vi "PickOffensiveRobots_v2.vi"(0 "object in":refnum<class "Game.lvclass">, 2 "GameRef":refnum<data-value>, 5 "error in (no error)":errorcluster) -> (14 "object out":refnum<class "Game.lvclass">, 19 "error out":errorcluster)   [LabVIEW 2023, in "Game.lvclass"]
uses:
  Game.lvclass
  Game.lvclass/Game.ctl
  Team_class/Team.lvclass/Team.ctl
  Team_class/Write RobotRef.vi
  Ally_class/Ally.lvclass
  C:/Users/ebert/Documents/codes/SSL/repo/SSL_AI/Team_class/Team.lvclass
  NewSTP/NewPlays/Play_v2_class/Play_v2.lvclass
  NewSTP/Playbook_v2_class/Playbook_v2.lvclass
panel:
  out "FPS":dbl
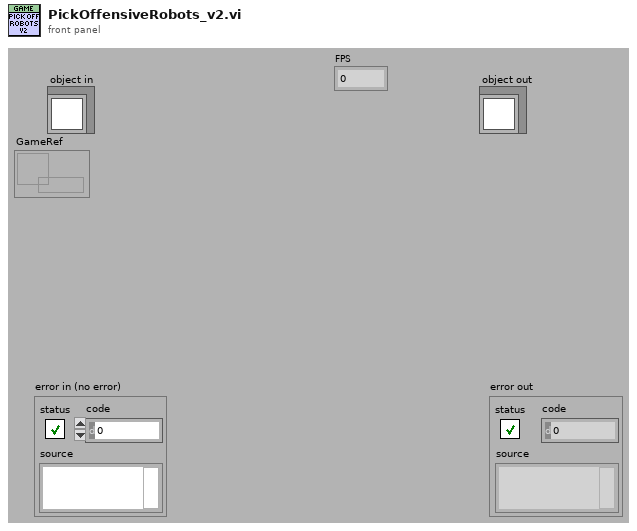
[diagram p1: front panel]
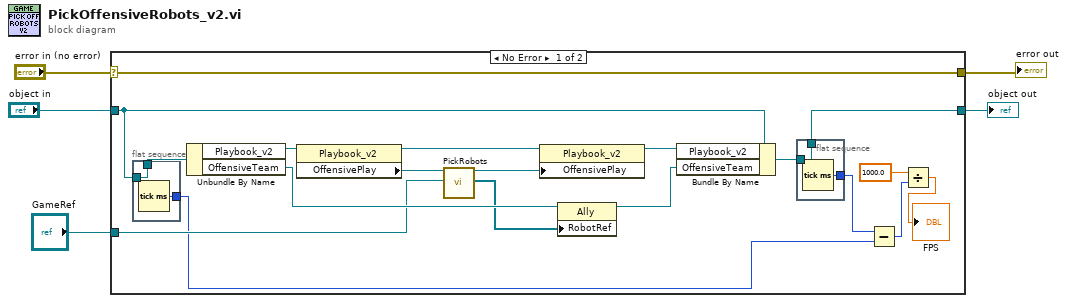
[diagram p0: block diagram]
diagram:
  n1 = case shown="No Error" "error in (no error)" {
    selector: "error in (no error)" -> [w24 w30]
    tunnel: [w24 w30] -> w4
    tunnel: [w11 w29] -> w2
    tunnel: "object in" -> [w14 w29]
    tunnel: "GameRef" -> [w15 _]
    frame No Error {
      n2 = flat-sequence {
        tunnel: w14 -> [w28]
        tunnel: [w28] -> w13
        tunnel: [w27] -> w9
        frame #0 {
          n3 = Tick Count (ms)() -> (millisecond timer value=w27:u32)
        }
      }
      n4 = Unbundle By Name(w13) -> ("Playbook_v2"=w23:refnum<class "Playbook_v2.lvclass">, "OffensiveTeam"=w21:refnum<class "Ally.lvclass">)
      n5 = property class="Playbook_v2"(reference=w23) -> (reference out=w19:refnum<class "Playbook_v2.lvclass">, "OffensivePlay"=w22:refnum<class "Play_v2.lvclass">)  [unwired: 1 in, 1 out]
      n6 = call-dynamic "PickRobots.vi"("object in"=w22, "GameRef"=w15) -> ("object out"=w18:refnum<class "Play_v2.lvclass">, "Robots"=w20:refnum<class "Robot.lvclass">[])  [unwired: 15 in, 1 out]
      n7 = property class="Playbook_v2"(reference=w19, "OffensivePlay"=w18) -> (reference out=w17:refnum<class "Playbook_v2.lvclass">)  [unwired: 1 in, 1 out]
      n8 = property class="Ally"(reference=w21, "RobotRef"=w20) -> (reference out=w16:refnum<class "Ally.lvclass">)  [unwired: 1 in, 1 out]
      n9 = Bundle By Name(cluster=w14, "Playbook_v2"=w17, "OffensiveTeam"=w16) -> (w12:refnum<class "Game.lvclass">)
      n10 = flat-sequence {
        tunnel: w12 -> [w26]
        tunnel: [w26] -> w11
        tunnel: [w25] -> w10
        frame #0 {
          n11 = Tick Count (ms)() -> (millisecond timer value=w25:u32)
        }
      }
      n12 = Subtract(x=w10, y=w9) -> (x-y=w7:u32)
      n13 = Divide(x=1000.0, y=w7) -> (x/y=→"FPS":dbl)
    }
    frame Error {
    }
  }
  "error out" <- w4
  "object out" <- w2
